vi "TractionControl_SubVI.vi"(0 "Drive Spd High Byte":u8, 1 "Target Slip":dbl, 5 "Drive Spd Low Byte":u8, 9 "Ground Spd High Byte":u8, 11 "Ground Spd Low Byte":u8) -> (4 "Drive Speed (mph)":dbl, 6 "Ground Speed (mph)":dbl, 8 "Calculated Slip":dbl, 13 "Drive Speed vs Ground Speed":cluster{dbl, dbl}(graph), 14 "Calculated Slip vs Target Slip":cluster{dbl, dbl}(graph))   [LabVIEW 2012]
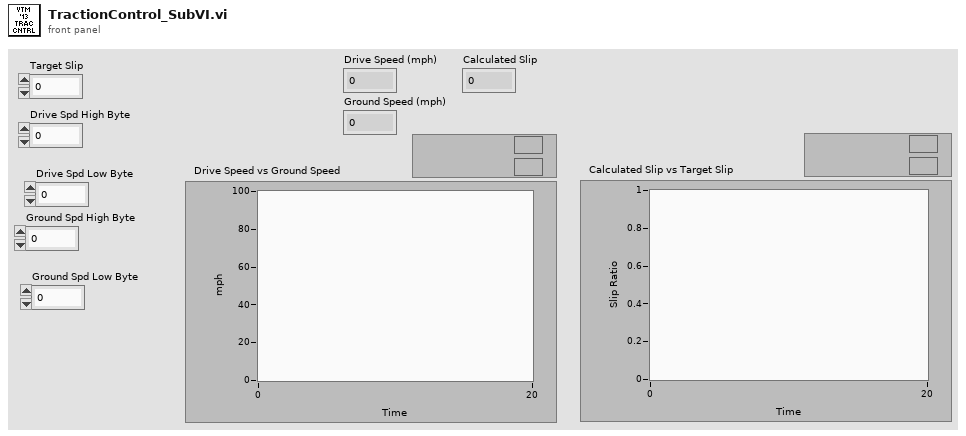
[diagram p1: front panel]
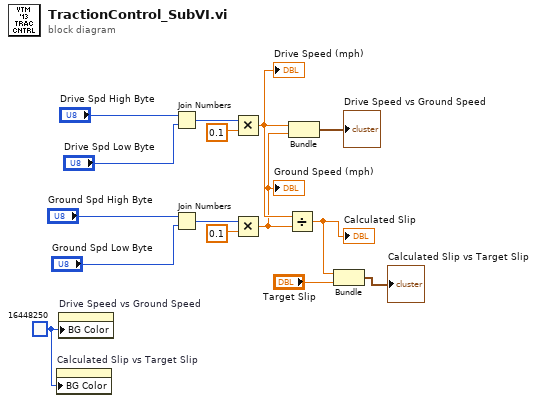
[diagram p0: block diagram]
diagram:
  w1 = u32 16448250
  n1 = property on="Calculated Slip vs Target Slip" class="WFChart (strict)"("BG Color"=w1) -> ()  [unwired: 2 in, 2 out]
  n2 = property on="Drive Speed vs Ground Speed" class="WFChart (strict)"("BG Color"=w1) -> ()  [unwired: 2 in, 2 out]
  n3 = Join Numbers(hi="Drive Spd High Byte", lo="Drive Spd Low Byte") -> ((hi.lo)=w11:u16)
  n4 = Join Numbers(hi="Ground Spd High Byte", lo="Ground Spd Low Byte") -> ((hi.lo)=w10:u16)
  n5 = Multiply(x=w11, y=0.1) -> (x*y=w6:dbl)
  "Drive Speed (mph)" <- w6
  n6 = Multiply(x=w10, y=0.1) -> (x*y=w5:dbl)
  "Ground Speed (mph)" <- w5
  n7 = Divide(x=w6, y=w5) -> (x/y=w4:dbl)
  "Calculated Slip" <- w4
  n8 = Bundle(w6, w5) -> (→"Drive Speed vs Ground Speed":cluster{dbl, dbl})  [unwired: 1 in]
  n9 = Bundle(w4, "Target Slip"="Target Slip") -> (→"Calculated Slip vs Target Slip":cluster{dbl, "Target Slip":dbl})  [unwired: 1 in]
